vi "Conversion.vi"(1 "String 3":string, 2 "String":string) -> (0 "Numeric":dbl)   [LabVIEW 2018]
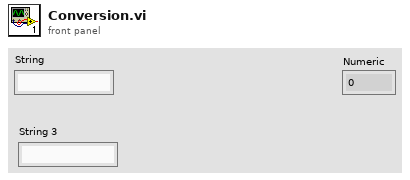
[diagram p1: front panel]
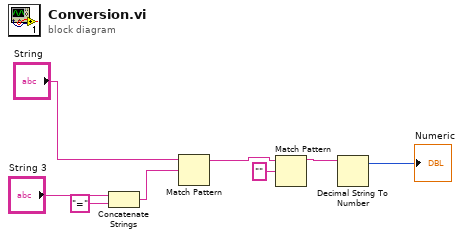
[diagram p0: block diagram]
diagram:
  n1 = Concatenate Strings("String 3", "=" ("string")) -> (w5:string)
  n2 = Match Pattern(string="String", regular expression=w5) -> (before substring=w3:string)  [unwired: 1 in, 3 out]
  n3 = Match Pattern(string=w3, regular expression="") -> (before substring=w2:string)  [unwired: 1 in, 3 out]
  n4 = Decimal String To Number(string=w2) -> (offset past number=→"Numeric":i32)  [unwired: 2 in, 1 out]
